vi "Configure Math Channel.vi"(5 "Channel (T: Enable)":bool=TRUE, 8 "error in (no error)":errorcluster, 9 "Source (0: Channel 1)":u16(ring) items=["Channel 1", "Channel 2", "Channel 3", "Channel 4", "Add", "Subtract", "Multiply"], 10 "Operation (0: Subtract)":u16(ring) items=["Subtract", "Multiply", "Integrate", "Differentiate", "FFT"], 11 "VISA resource name":refnum<visa-resource-name>) -> (0 "error out":errorcluster, 3 "VISA resource name out":refnum<visa-resource-name>)   [LabVIEW 2017, in "Agilent 6000 Series.lvlib"]
doc: "This VI configures the properties that control the math channel. These properties are the sources and operation.\n\n<B>Note:</B>\n(1) This VI has been obsoleted from the driver and is included for compatibility with existing applications. New applications should use the <B>Configure Math Function</B> VI."
uses:
  <instrlib>/Agilent 6000 Series/Agilent 6000 Series.lvlib
panel:
  # "Note:\nThis VI has been obsoleted from the driver and is included for\ncompatibility with existing applications. New applications should use\nthe Configure Math Function VI."
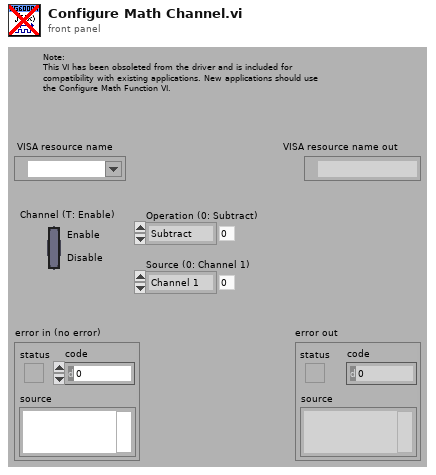
[diagram p1: front panel]
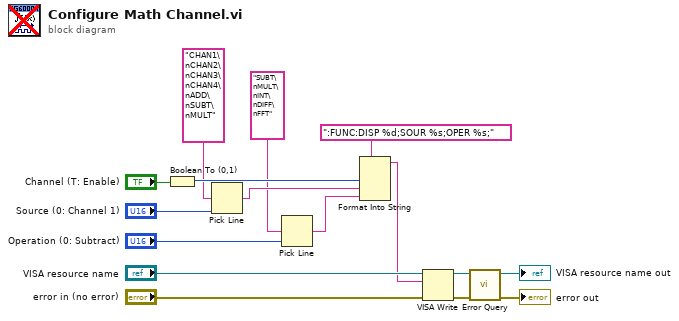
[diagram p0: block diagram]
diagram:
  n1 = Boolean To (0,1)(Boolean="Channel (T: Enable)") -> (0, 1=w7:i16)
  n2 = Pick Line(multi-line string="CHAN1\nCHAN2\nCHAN3\nCHAN4\nADD\nSUBT\nMULT", line index="Source (0: Channel 1)") -> (output string=w4:string)  [unwired: 1 in]
  n3 = Pick Line(multi-line string="SUBT\nMULT\nINT\nDIFF\nFFT", line index="Operation (0: Subtract)") -> (output string=w1:string)  [unwired: 1 in]
  n4 = Format Into String(format string=":FUNC:DISP %d;SOUR %s;OPER %s;", w7, w4, w1) -> (resulting string=w9:string)  [unwired: 2 in, 1 out]
  n5 = VISA Write(VISA resource name="VISA resource name", write buffer=w9, error in (no error)="error in (no error)") -> (VISA resource name out=w12:refnum<visa-resource-name>, error out=w11:errorcluster)  [unwired: 1 out]
  n6 = call <instrlib>:"Error Query.vi"("error in (no error)"=w11, "VISA resource name"=w12) -> ("error out"=→"error out":errorcluster, "VISA resource name out"=→"VISA resource name out":refnum<visa-resource-name>)  [unwired: 6 in, 2 out]
